vi "HapticSTM_nano.vi"() -> ()   [LabVIEW 2017]
uses:
  Program Files/National Instruments/LabVIEW 2019/user.lib/HapticSTM/HapticSTM.lvlib
  SubVIs/GlobalClicksHeight_nano.vi
  <vilib>/sound2/lvsound2.llb/Sampling Mode.ctl
  <vilib>/sound2/lvsound2.llb/Sound Data Format.ctl
  <vilib>/sound2/lvsound2.llb/Sound Output Set Volume (Single).vi
  <vilib>/sound2/lvsound2.llb/Sound Output Write (DBL Single).vi
  Program Files/National Instruments/LabVIEW 2019/user.lib/Nanonis Prog Interface V5/Nanonis Prog Interface.lvlib
panel:
  in  "Z Write?":bool
  in  "Sound\nActivation":bool=TRUE
  in  "Sensitivity":dbl=1.0 format="%.1f"
  in  "Volume":dbl(slide)=50.0 scale=0.0..100.0
  in  "Device ID":u32
  out "function return":i32
  in  "Surface Shift (in)":dbl format="%.1f"
  in  "Scaling?":bool
  out "Setpoint (pA)":dbl
  in  "Maximum (pA)":dbl=9000.0
  out "Filtered Current (pA)":dbl format="%.1f"
  out "Current (pA)":dbl format="%.1f"
  out "Oy":dbl
  out "Ox":dbl
  out "W":dbl
  out "H":dbl
  out "Z Write":dbl format="%^.1e"
  out "Z Read":dbl format="%^#.1e"
  in  "Planing?":bool
  in  "Plunge Depth (pA)":dbl=280.0 format="%.1f"
  out "Button":bool
  out "Vy":dbl format="%.1f"
  out "Vz":dbl format="%.1f"
  out "Vx":dbl format="%.1f"
  out "Fy":dbl format="%.1f"
  out "Fz":dbl format="%.1f"
  out "Fx":dbl format="%.1f"
  out "phi":dbl format="%.1f"
  out "psi":dbl format="%.1f"
  out "theta":dbl format="%.1f"
  out "x":dbl format="%.1f"
  out "y":dbl format="%.1f"
  out "z":dbl format="%0.1f"
  out "Height":dbl format="%^.1e"
  in  "Hardness":dbl=1.0 format="%.1f"
  in  "Mode":u16(ring) items=["Log w/ Exp Z", "Log w/ Lin Z"]
  in  "Reset Clicks":bool
  out "Clicks":i32
  in  "STOP":bool
  in  "START":bool
  out "Seq":i32
  out "SeqString":string
  out "Raw and Scaled Z Positions":cluster{dbl, "Y":dbl}(graph)
  out "Scaled Force and Current":T1(graph)
  # "Super Ultra Mega Haptic STM Controller 3000"
  # "Nanonis"
  # "Small"
  # "Large"
  # "Addons"
  # "Sound Module"
  # "Current"
  # "Frame"
  # "Z Controller"
  # "No"
  # "Yes"
  # "Haptic Pen"
  # "Position"
  # "Force"
  # "Angles"
  # "Velocity"
  # "Surface"
  # "Clicks"
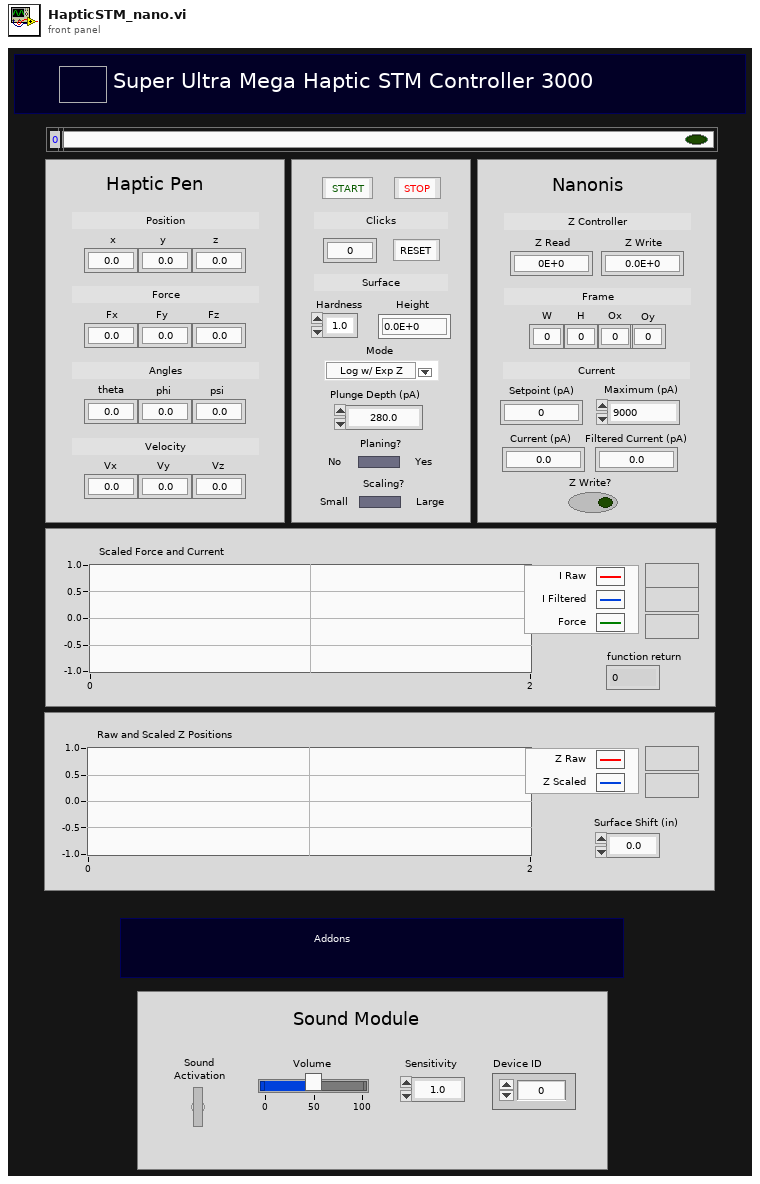
[diagram p1: front panel]
types:
  T1 = cluster{"Current (pA)":sgl, "Filtered Current (pA)":dbl, dbl}
  T2 = typedef "Sound Data Format.ctl" = cluster{"sample rate (S/s)":dbl, "number of channels":i32, "bits per sample":i32}
  T3 = typedef "Sampling Mode.ctl" = i32
  T4 = typedef "Sound Output Task ID.ctl" = u32
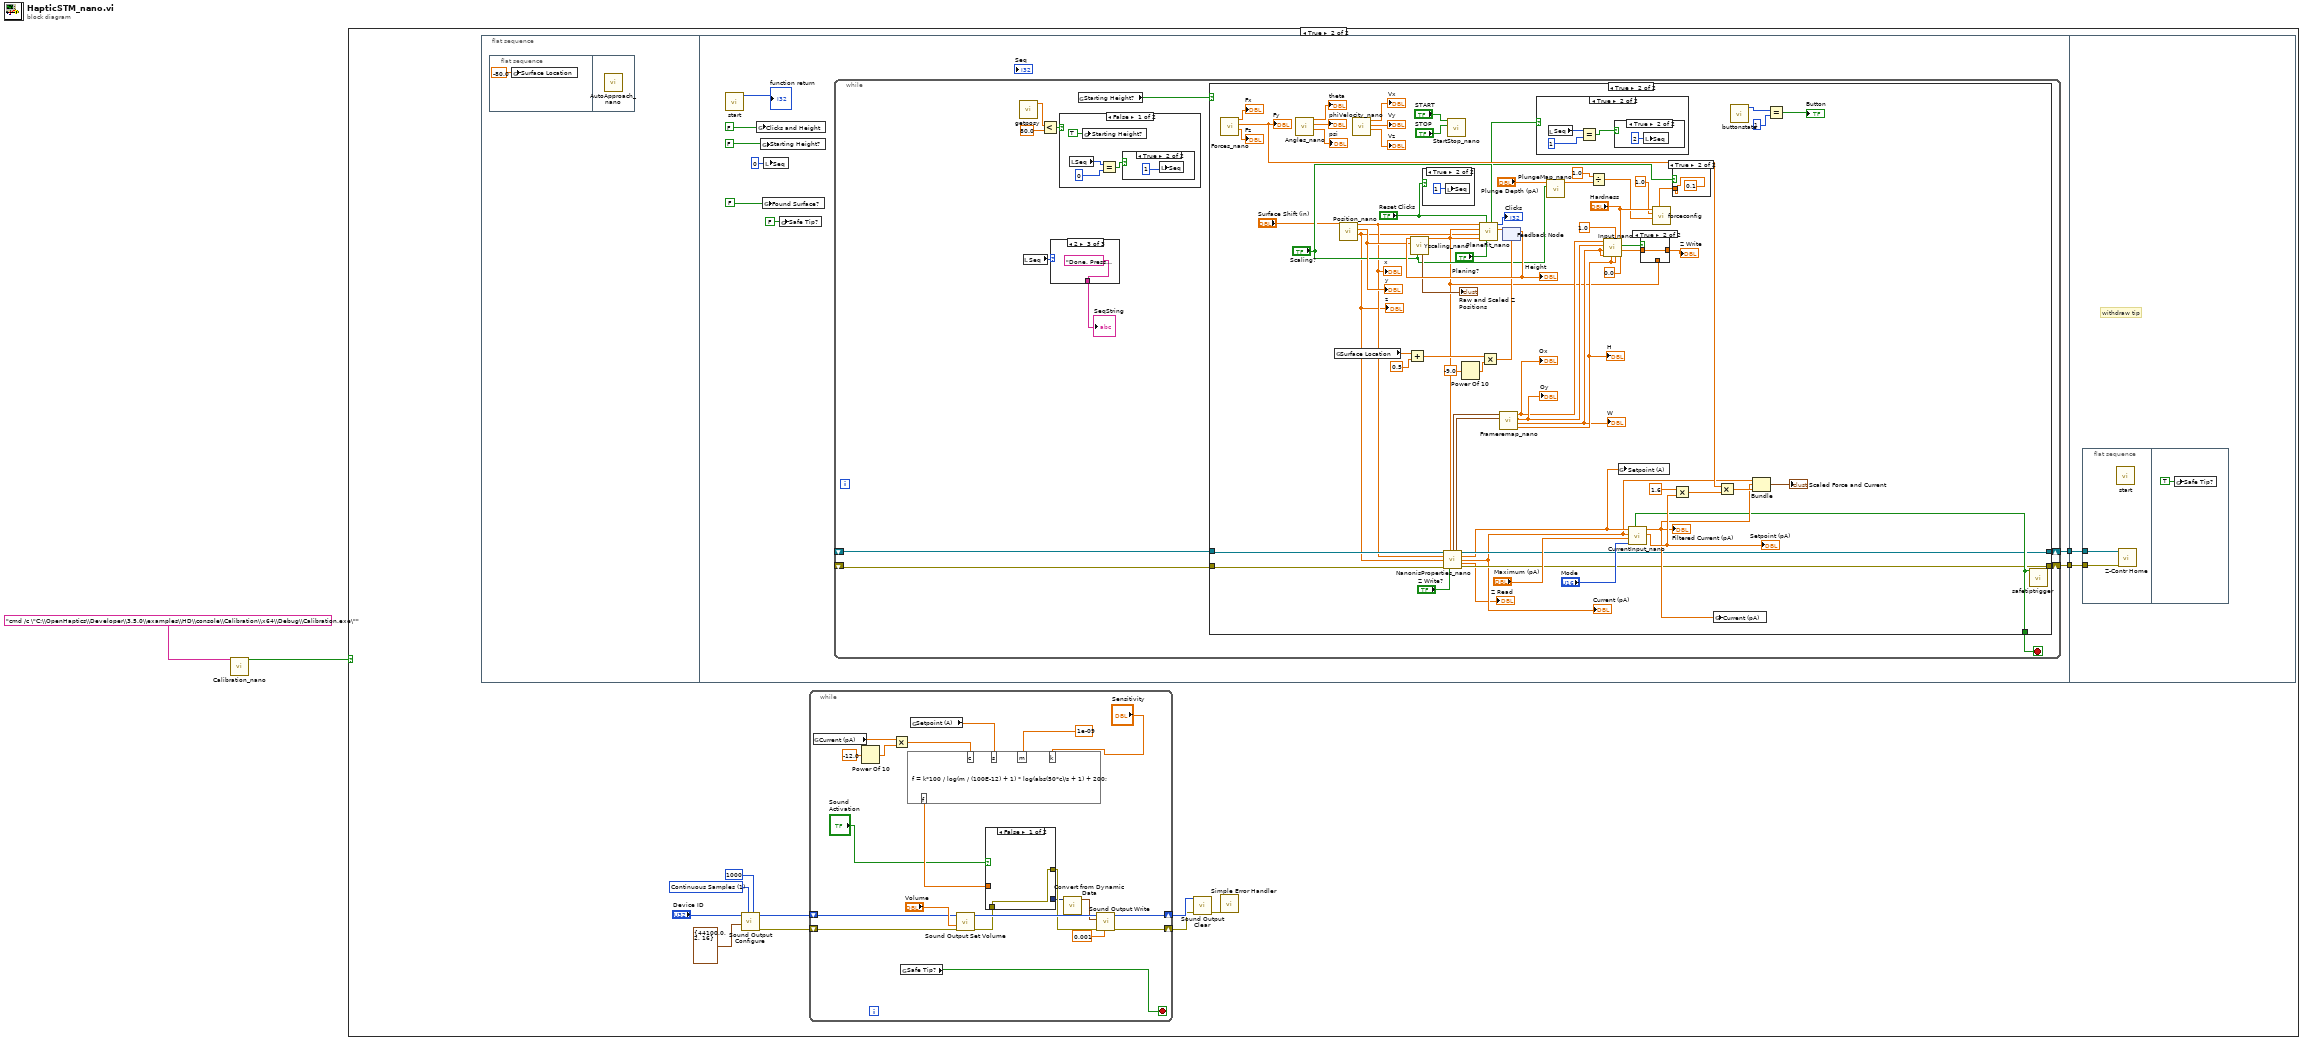
[diagram p0: block diagram]
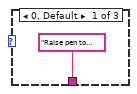
[diagram p3: hidden frame]
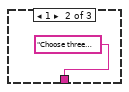
[diagram p4: hidden frame]
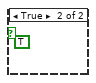
[diagram p6: hidden frame]
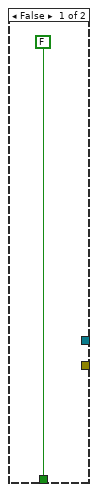
[diagram p7: hidden frame]
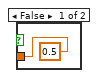
[diagram p8: hidden frame]
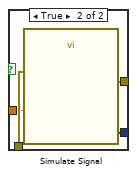
[diagram p13: hidden frame]
diagram:
  n1 = call "Calibration_nano.vi"("command line"="cmd /c \"C:\\OpenHaptics\\Developer\\3.5.0\\examples\\HD\\console\\Calibration\\x64\\Debug\\Calibration.exe\"") -> ("Calibration Complete?"=w2:bool)  [unwired: 10 in]
  n2 = case shown="True" w2 {
    frame False {
    }
    frame True {
      w12 = T3 1 items=["Finite Samples", "Continuous Samples"] ("sample mode")
      n3 = flat-sequence {
        tunnel: [w16] -> w4
        tunnel: [w15] -> w3
        tunnel: w4 -> [w121]
        tunnel: w3 -> [w120]
        frame #0 {
          n4 = flat-sequence {
            frame #0 {
              n5 = global write "GlobalClicksHeight_nano.vi" "Surface Location"(-80.0 ("Surface Location")) -> ()
            }
            frame #1 {
              n6 = call "AutoApproach_nano.vi"() -> ()  [unwired: 12 in]
            }
          }
        }
        frame #1 {
          n7 = call "start.vi"() -> ("function return"=→"function return":i32)  [unwired: 11 in]
          n8 = global write "GlobalClicksHeight_nano.vi" "Clicks and Height"(FALSE ("Clicks and Height")) -> ()
          n9 = global write "GlobalClicksHeight_nano.vi" "Starting Height?"(FALSE ("Clicks and Height")) -> ()
          n10 = global write "GlobalClicksHeight_nano.vi" "Found Surface?"(FALSE ("Clicks and Height")) -> ()
          n11 = local write "Seq"(0 ("Seq")) -> ()
          n12 = global write "GlobalClicksHeight_nano.vi" "Safe Tip?"(FALSE ("Safe Tip?")) -> ()
          n13 = while {
            shift-right: [w26] -> w15
            shift-left: _ -> [w23]
            shift-right: [w24] -> w16
            shift-left: _ -> [w25]
            stop <- w27 stop-if-true
            n14 = call "getposy.vi"() -> ("function return"=w33:dbl)  [unwired: 11 in]
            n15 = local read "Seq"() -> (w29:i32)
            n16 = Less?(x=w33, y=80.0) -> (x < y?=w31:bool)
            n17 = case shown="2" w29 {
              tunnel: ["Raise pen to begin." "Choose three points, then raise the arm to plane." "Done. Press 'STOP' to stop at anytime."] -> w28
              frame 0, Default {
              }
              frame 1 {
              }
              frame 2 {
              }
            }
            "SeqString" <- w28
            n18 = case shown="False" w31 {
              frame False {
                n19 = local read "Seq"() -> (w39:i32)
                n20 = global write "GlobalClicksHeight_nano.vi" "Starting Height?"(TRUE ("Starting Height?")) -> ()
                n21 = Equal?(x=w39, y=0) -> (x = y?=w37:bool)
                n22 = case shown="True" w37 {
                  frame False {
                  }
                  frame True {
                    n23 = local write "Seq"(1 ("Seq")) -> ()
                  }
                }
              }
              frame True {
                (unwired) TRUE ("Clicks and Height")
              }
            }
            n24 = global read "GlobalClicksHeight_nano.vi" "Starting Height?"() -> (w30:bool)
            n25 = case shown="True" w30 {
              tunnel: [FALSE ("Current Maxed?") w57] -> w27
              tunnel: w23 -> [_ w55]
              tunnel: [_ w54] -> w26
              tunnel: w25 -> [_ w53]
              tunnel: [_ w52] -> w24
              frame False {
              }
              frame True {
                n26 = call "Forces_nano.vi"() -> ("Fz"=→"Fz":dbl, "Fy"=w96:dbl, "Fx"=→"Fx":dbl)  [unwired: 9 in]
                "Fy" <- w96
                n27 = call "Angles_nano.vi"() -> ("psi"=→"psi":dbl, "phi"=→"phi":dbl, "theta"=→"theta":dbl)  [unwired: 9 in]
                n28 = global read "GlobalClicksHeight_nano.vi" "Surface Location"() -> (w66:dbl)
                n29 = call "Position_nano.vi"("Shift"="Surface Shift (in)") -> ("Z"=w47:dbl, "Y"=w92:dbl, "X"=w48:dbl)  [unwired: 8 in]
                "x" <- w48
                "y" <- w92
                "z" <- w47
                n30 = call "Velocity_nano.vi"() -> ("VZ"=→"Vz":dbl, "VY"=→"Vy":dbl, "VX"=→"Vx":dbl)  [unwired: 9 in]
                n31 = Add(x=w66, y=0.5) -> (x+y=w63:dbl)
                n32 = case shown="True" "Reset Clicks" {
                  frame False {
                  }
                  frame True {
                    n33 = local write "Seq"(1 ("Seq")) -> ()
                  }
                }
                n34 = call "StartStop_nano.vi"("STOP"="STOP", "START"="START") -> ()  [unwired: 10 in]
                n35 = Power Of 10(x=-9.0) -> (10^x=w62:dbl)
                n36 = Multiply(x=w63, y=w62) -> (x*y=w64:dbl)
                n37 = feedback #1(w64) -> (w98:dbl)
                "Height" <- w98
                n38 = call "Yscaling_nano.vi"("Scaling?"="Scaling?", "Y"=w92, "Plane Height"=w98) -> ("y scaled (m)"=w49:dbl, "Zpos Graph (nm)"=→"Raw and Scaled Z Positions":cluster{dbl, "function return":dbl})  [unwired: 7 in]
                n39 = call "NanonisProperties_nano.vi"("Application reference"=w53, "Z Write (m)"=w49, "X pen (nm)"=w48, "Z pen (nm)"=w47, "Error in"=w55, "Z Write?"="Z Write?") -> ("Frame Size (m)"=w51:cluster{"Width":sgl, "Height":sgl}, "Frame Origin (m)"=w50:cluster{"Xc":sgl, "Yc":sgl}, "Application ref out"=w52:refnum<vi>, "Setpoint (A)"=w46:sgl, "Current (pA)"=w45:sgl, "Z Read (m)"=→"Z Read":sgl, "error out"=w54:errorcluster)  [unwired: 3 in]
                "Current (pA)" <- w45
                n40 = call "PlaneFit_nano.vi"("Planing y/n?"="Planing?", "Reset Clicks"="Reset Clicks", "Y PEN"=w49, "Z"=w47, "Nano Z"=w49, "X"=w48) -> ("Plane Height (m)"=w99:dbl, "Clicks"=→"Clicks":i32, "Planing Done?"=w85:bool)  [unwired: 3 in]
                n41 = call "Frameremap_nano.vi"("Frame Origin (m)"=w50, "Frame Size (m)"=w51) -> ("FH (nm)"=w76:dbl, "FW (nm)"=w75:dbl, "Z Origin (nm)"=w74:dbl, "X Origin (nm)"=w73:dbl)  [unwired: 6 in]
                "H" <- w76
                "W" <- w75
                "Ox" <- w73
                "Oy" <- w74
                n42 = feedback-in #1(w99) -> ()
                n43 = case shown="True" w85 {
                  frame False {
                  }
                  frame True {
                    n44 = local read "Seq"() -> (w118:i32)
                    n45 = Equal?(x=w118, y=1) -> (x = y?=w116:bool)
                    n46 = case shown="True" w116 {
                      frame False {
                      }
                      frame True {
                        n47 = local write "Seq"(2 ("Seq")) -> ()
                      }
                    }
                  }
                }
                n48 = call "PlungeMap_nano.vi"("Scaling?"="Scaling?", "Input (pA)"="Plunge Depth (pA)") -> ("output"=w67:dbl)  [unwired: 9 in]
                n49 = Divide(x=1.0, y=w67) -> (x/y=w77:dbl)
                n50 = call "Input_nano.vi"("Current * 10^input"=0.0, "Sensitivity"="Hardness", "Scopez"=w76, "Drag"=1.0, "FH"=w76, "FW"=w75, "Scopex"=w75, "Z origin"=w74, "X origin"=w73) -> ("Scaled Current"=w79:dbl, "feedback"=w81:bool)  [unwired: 1 in]
                n51 = global write "GlobalClicksHeight_nano.vi" "Setpoint (A)"(w46) -> ()
                n52 = call "CurrentInput_nano.vi"("Mode"="Mode", "Maximum (pA)"="Maximum (pA)", "Current (pA)"=w45, "Setpoint (A)"=w46) -> ("Setpoint (pA)"=w69:dbl, "Filtered Current (pA)"=w60:dbl, "Safetip?"=w57:bool)  [unwired: 5 in]
                "Filtered Current (pA)" <- w60
                "Setpoint (pA)" <- w69
                n53 = case shown="True" w81 {
                  tunnel: [w113 w114] -> w80
                  tunnel: w79 -> [_ w114]
                  tunnel: w49 -> [w113 _]
                  frame False {
                  }
                  frame True {
                  }
                }
                "Z Write" <- w80
                n54 = case shown="True" "Scaling?" {
                  tunnel: [0.5 0.1] -> w59
                  frame False {
                  }
                  frame True {
                  }
                }
                n55 = call "forceconfig.vi"("spc"=w59, "c"=w77, "b"=1.0, "a"="Hardness") -> ()  [unwired: 8 in]
                n56 = Multiply(x=1.6 ("y"), y=w69) -> (x*y=w93:dbl)
                n57 = global write "GlobalClicksHeight_nano.vi" "Current (pA)"(w60) -> ()
                n58 = Multiply(x=w96, y=w93) -> (x*y=w95:dbl)
                n59 = call "buttonstate.vi"() -> ("function return"=w91:i32)  [unwired: 11 in]
                n60 = Bundle("Current (pA)"=w45, "Filtered Current (pA)"=w60, w95) -> (→"Scaled Force and Current":T1)  [unwired: 1 in]
                n61 = Equal?(x=w91, y=1) -> (x = y?=→"Button":bool)
                n62 = call "safetiptrigger.vi"("triggered"=w57) -> ()  [unwired: 11 in]
              }
            }
          }
        }
        frame #2 {
          # "withdraw tip"
          n63 = flat-sequence {
            tunnel: w121 -> [w123]
            tunnel: w120 -> [w122]
            frame #0 {
              n64 = call "start.vi"() -> ()  [unwired: 11 in, 1 out]
              n65 = call <userlib>:"Z-Contr Home.vi"("Error in (no error)"=w122, "Application ref in"=w123) -> ()  [unwired: 8 in, 2 out]
            }
            frame #1 {
              n66 = global write "GlobalClicksHeight_nano.vi" "Safe Tip?"(TRUE ("Safe Tip?")) -> ()
            }
          }
        }
      }
      n67 = call <vilib>:"Sound Output Configure.vi"("number of samples/ch"=1000 ("Number of Samples/ch"), "sample mode"=w12, "sound format"=T2 {"sample rate (S/s)"=44100.0, "number of channels"=2, "bits per sample"=16} ("Sound Format"), "device ID"="Device ID") -> ("error out"=w8:errorcluster, "task ID"=w9:T4)  [unwired: 6 in]
      n68 = while {
        shift-right: [w137] -> w7
        shift-left: w9 -> [w139]
        shift-right: [w136] -> w6
        shift-left: w8 -> [w138]
        stop <- w126 stop-if-true
        n69 = global read "GlobalClicksHeight_nano.vi" "Current (pA)"() -> (w129:dbl)
        n70 = Power Of 10(x=-12.0) -> (10^x=w131:dbl)
        n71 = Multiply(x=w129, y=w131) -> (x*y=w128:dbl)
        n72 = global read "GlobalClicksHeight_nano.vi" "Safe Tip?"() -> (w126:bool)
        n73 = global read "GlobalClicksHeight_nano.vi" "Setpoint (A)"() -> (w133:dbl)
        n74 = formula code="f = k*100 / log(m / (100E-12) + 1) * log(abs(50*c)/s + 1) + 200;"("c"=w128, "m"=1e-09 ("input variable"), "s"=w133, "k"="Sensitivity") -> ("f"=w132:dbl)
        n75 = call-poly <vilib>:"Sound Output Set Volume.vi"("error in (no error)"=w138, "volume"="Volume", "task ID"=w139) -> ("error out"=w142:errorcluster, "task ID out"=w145:T4)  [unwired: 7 in]
        n76 = case shown="False" "Sound\nActivation" {
          tunnel: w142 -> [w146 w150]
          tunnel: [w146 w149] -> w141
          tunnel: [_ w148] -> w140
          tunnel: w132 -> [_ w147]
          frame False {
          }
          frame True {
            n77 = call "Simulate Signal"("Frequency"=w147, "error in (no error)"=w150) -> ("Sine"=w148:dynamicdata, "error out"=w149:errorcluster)  [unwired: 12 in]
          }
        }
        n78 = call "Convert from Dynamic Data"("Dynamic Data Type"=w140) -> ("Waveform"=w143:waveform(dbl))  [unwired: 3 in]
        n79 = call-poly <vilib>:"Sound Output Write.vi"("timeout (sec)"=0.001, "error in (no error)"=w141, "data"=w143, "task ID"=w145) -> ("error out"=w136:errorcluster, "task ID out"=w137:T4)  [unwired: 6 in]
      }
      n80 = call <vilib>:"Sound Output Clear.vi"("error in (no error)"=w6, "task ID"=w7) -> ("error out"=w11:errorcluster)  [unwired: 9 in]
      n81 = call <vilib>:"Simple Error Handler.vi"("error in (no error)"=w11) -> ()  [unwired: 4 in, 5 out]
    }
  }
